vi "PT100.vi"(1 "Resistance, (Ohm)":dbl) -> (0 "Temperature, (K)":dbl)   [LabVIEW 2016]
panel:
  out "String":string="Pt100"
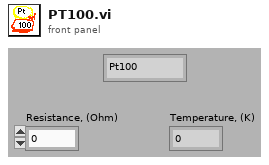
[diagram p1: front panel]
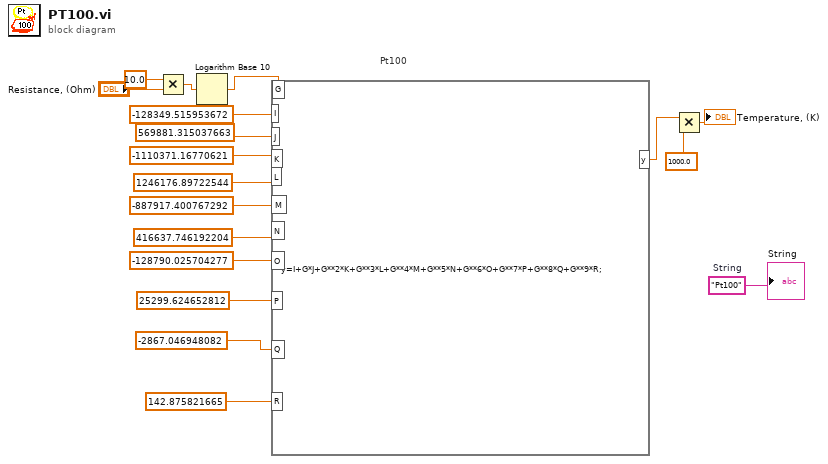
[diagram p0: block diagram]
diagram:
  w6 = "Pt100"  # String
  # "Pt100"
  n1 = Multiply(x=10.0, y="Resistance, (Ohm)") -> (x*y=w4:dbl)
  n2 = Logarithm Base 10(1:w4) -> (0:w18:dbl)
  n3 = formula code="y=I+G*J+G**2*K+G**3*L+G**4*M+G**5*N+G**6*O+G**7*P+G**8*Q+G**9*R;"("G"=w18, "I"=-128349.515953672 ("input variable"), "L"=1246176.89722544 ("input variable"), "M"=-887917.400767292 ("input variable"), "O"=-128790.025704277 ("input variable"), "Q"=-2867.046948082 ("input variable"), "R"=142.875821665 ("input variable"), "P"=25299.624652812 ("input variable"), "N"=416637.746192204 ("input variable"), "J"=569881.315037663 ("input variable"), "K"=-1110371.16770621 ("input variable")) -> ("y"=w17:dbl)
  n4 = Multiply(x=w17, y=1000.0) -> (x*y=→"Temperature, (K)":dbl)
  "String" <- w6
